vi "front_panel.vi"() -> ()   [LabVIEW 2017]
panel:
  out "Indicator4":string
  out "Indicator3":string
  out "Indicator2":string
  out "Indicator1":string
  in  "Reset Button":bool
  in  "Stop Button":bool
  in  "OK Button":bool
  in  "Start Button":bool
  in  "Data":string
  out "Box5":bool
  out "Box4":bool
  out "Box3":bool
  out "Box2":bool
  out "Box1":bool
  in  "Right Buttons":cluster{"Button 3":bool, "Button 4":bool}
  in  "Left Buttons":cluster{"Button 1":bool, "Button 2":bool}
  out "Screen":string
  # "Parcel Locker"
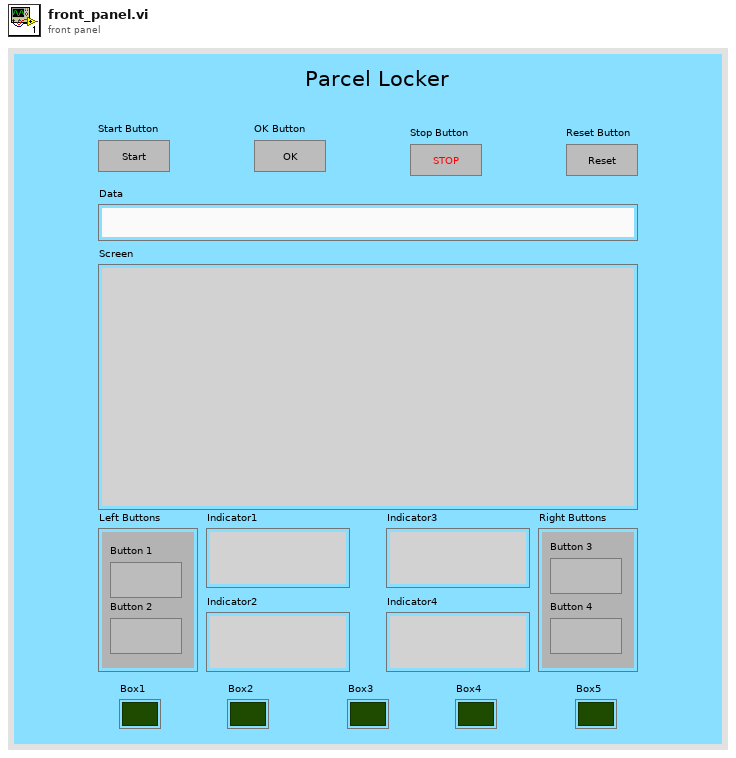
[diagram p1: front panel]
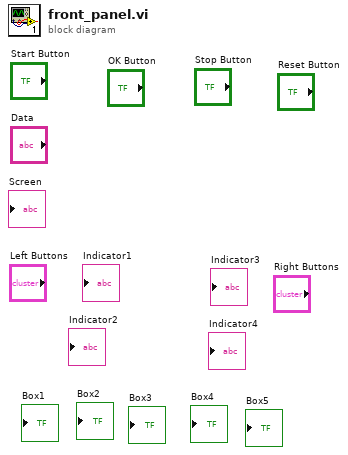
[diagram p0: block diagram]
diagram:
